vi "name test.vi"() -> ()   [LabVIEW 2017, in "Communication.lvlib"]
uses:
  Communication/Communication.lvlib
panel:
  out "before substring":string
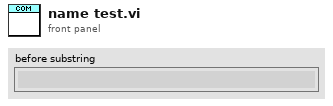
[diagram p1: front panel]
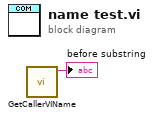
[diagram p0: block diagram]
diagram:
  n1 = call "GetCallerVIName.vi"() -> ("before substring"=→"before substring":string)  [unwired: 11 in]
